vi "Separate Inline and Async.vi"(8 "error in (no error)":errorcluster, 11 "Transfer Groups":refnum<class "Transfer Group.lvclass">[](array[class])) -> (0 "error out":errorcluster, 2 "Async Transfer Groups":refnum<class "Transfer Group.lvclass">[](array[class]), 3 "Inline Transfer Groups":refnum<class "Transfer Group.lvclass">[](array[class]))   [LabVIEW 2021, in "DSF Core.lvlib" / "Transfer Group.lvclass"]
uses:
  Transfer Group.lvclass
  Transfer Group.lvclass/Transfer Group.ctl
  Timing/Timing.lvclass/Timing.ctl
  Timing/Timing.lvclass
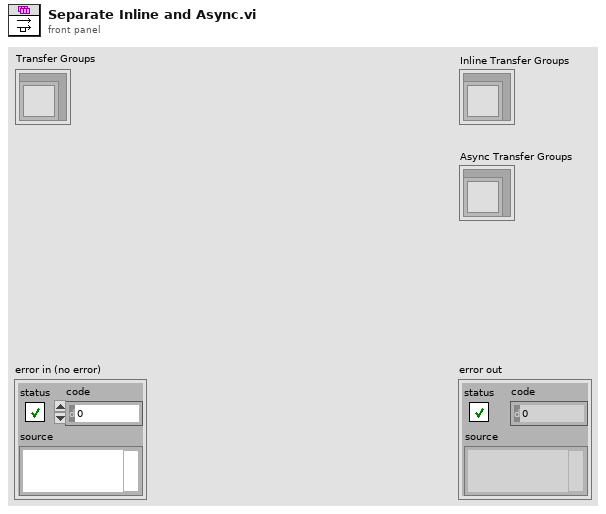
[diagram p1: front panel]
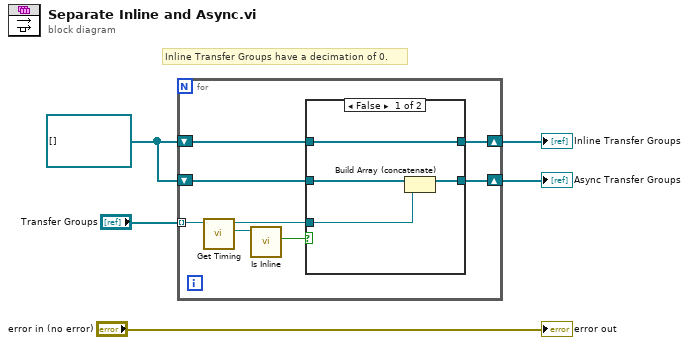
[diagram p0: block diagram]
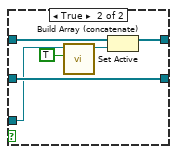
[diagram p2: hidden frame]
diagram:
  w3 = refnum<class "Transfer Group.lvclass">[] [] ("Transfer Groups")
  # "Inline Transfer Groups have a decimation of 0."
  n1 = for {
    tunnel: "Transfer Groups" -> [w13] mode=indexing
    shift-right: [w9] -> w2
    shift-left: w3 -> [w12]
    shift-right: [w8] -> w1
    shift-left: w3 -> [w10]
    n2 = call "Get Timing.vi"("Transfer Group in"=w13) -> ("Timing"=w7:refnum<class "Timing.lvclass">, "Transfer Group out"=w11:refnum<class "Transfer Group.lvclass">)  [unwired: 9 in]
    n3 = call "Is Inline.vi"("Timing in"=w7) -> ("inline?"=w6:bool)  [unwired: 9 in, 1 out]
    n4 = case shown="False" w6 {
      tunnel: w12 -> [w17 w22]
      tunnel: w11 -> [w16 w20]
      tunnel: w10 -> [w15 w23]
      tunnel: [w17 w21] -> w9
      tunnel: [w14 w23] -> w8
      frame False {
        n5 = Build Array (concatenate)(w15, w16) -> (w14:refnum<class "Transfer Group.lvclass">[])
      }
      frame True {
        n6 = call "Set Active.vi"("active"=TRUE, "Transfer Group in"=w20) -> ("Transfer Group out"=w19:refnum<class "Transfer Group.lvclass">)  [unwired: 9 in]
        n7 = Build Array (concatenate)(w22, w19) -> (w21:refnum<class "Transfer Group.lvclass">[])
      }
    }
  }
  "Inline Transfer Groups" <- w2
  "Async Transfer Groups" <- w1
  "error out" <- "error in (no error)"
